vi "Read Nested Viewable Enqueuers.vi"(11 "IViewManager in":refnum<class "IViewManager.lvclass">) -> (1 "Viewable Names":string[](array[string]), 2 "Nested Viewable Enqueuers":refnum<class "Message Enqueuer.lvclass">[](array[class]))   [LabVIEW 2015, in "IViewManager.lvlib" / "IViewManager.lvclass"]
uses:
  IViewManager.lvclass
  <vilib>/ActorFramework/Message Enqueuer/Message Enqueuer.lvclass
  IViewManager.lvclass/IViewManager.ctl
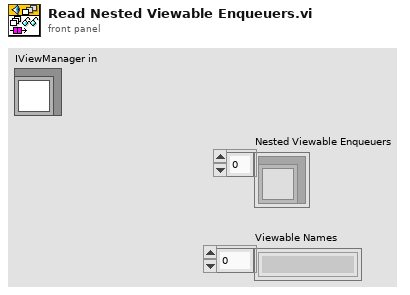
[diagram p1: front panel]
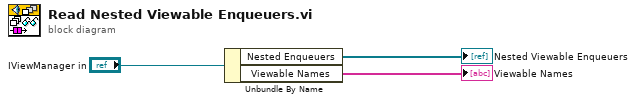
[diagram p0: block diagram]
diagram:
  n1 = Unbundle By Name("IViewManager in") -> ("Nested Enqueuers"=→"Nested Viewable Enqueuers":refnum<class "Message Enqueuer.lvclass">[], "Viewable Names"=→"Viewable Names":string[])
